vi "Record Log.vi"(7 "Record?":bool=TRUE, 8 "Error In":errorcluster, 10 "Data":string, 11 "Event":string) -> (0 "Error Out":errorcluster)   [LabVIEW 2019]
uses:
  <vilib>/Utility/file.llb/Write Delimited Spreadsheet (string).vi
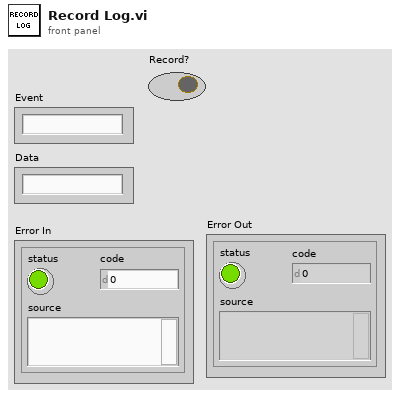
[diagram p1: front panel]
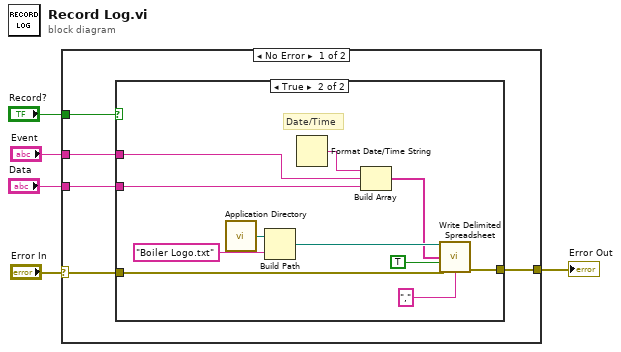
[diagram p0: block diagram]
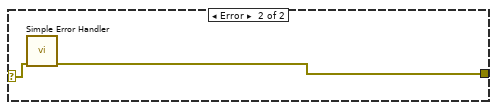
[diagram p3: hidden frame]
diagram:
  n1 = case shown="No Error" "Error In" {
    selector: "Error In" -> [w7 w24]
    tunnel: [w8 w23] -> w4
    tunnel: "Data" -> [w9 _]
    tunnel: "Event" -> [w10 _]
    tunnel: "Record?" -> [w6 _]
    frame No Error {
      n2 = case shown="True" w6 {
        tunnel: w10 -> [_ w18]
        tunnel: w9 -> [_ w17]
        tunnel: [w11 w14] -> w8
        tunnel: w7 -> [w11 w13]
        frame False {
        }
        frame True {
          # "Date/Time"
          n3 = call <vilib>:"Application Directory.vi"() -> ("Application Directory"=w21:path)
          n4 = Build Path(base path=w21, name or relative path="Boiler Logo.txt") -> (appended path=w15:path)
          n5 = Format Date/Time String() -> (date/time string=w19:string)  [unwired: 3 in]
          n6 = Build Array(w19, w18, w17) -> (w12:string[])
          n7 = call-poly <vilib>:"Write Delimited Spreadsheet.vi"("file path (dialog if empty)"=w15, "1D data"=w12, "append to file? (new file:F)"=TRUE, "error in (no error)"=w13, "delimiter (\\t)"="," ("delimiter (\\t)")) -> ("error out"=w14:errorcluster)  [unwired: 9 in, 1 out]
        }
      }
    }
    frame Error {
      n8 = call <vilib>:"Simple Error Handler.vi"("error in (no error)"=w24) -> ("error out"=w23:errorcluster)  [unwired: 4 in, 4 out]
    }
  }
  "Error Out" <- w4
